vi "TranslateTyping.vi"(11 "Cluster":T2) -> (2 "key":string)   [LabVIEW 2020]
uses:
  <vilib>/event_ctls.llb/eventvkey.ctl
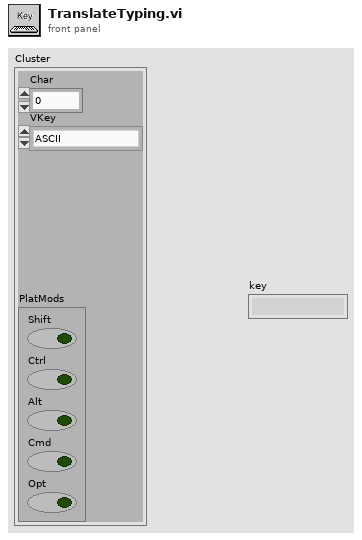
[diagram p1: front panel]
types:
  T1 = typedef "eventvkey.ctl" = enum16{"ASCII", "Enter", "Return", "Shift", "Ctrl", "Alt", "Cmd", "Opt", "Caps", "NumLock", "Clear", "Break", "Up", "Down", "Left", "Right", "Insert", "Delete", "Home", "End", "PageUp", "PageDown", "Escape", "Help", "Pause", "ScrollLock", "F1", "F2", "F3", "F4", "F5", "F6", "F7", "F8", "F9", "F10", "F11", "F12", "F13", "F14", "F15", "F16", "F17", "F18", "F19", "F20", "F21", "F22", "F23", "F24", "Play", "VolumeUp", "VolumeDown", "Mute", "Two Byte Char"}
  T2 = cluster{"Char":i16, "VKey":T1, "PlatMods":cluster{"Shift":bool, "Ctrl":bool, "Alt":bool, "Cmd":bool, "Opt":bool}}
  T3 = cluster{"Shift":bool, "Ctrl":bool, "Alt":bool, "Cmd":bool, "Opt":bool}
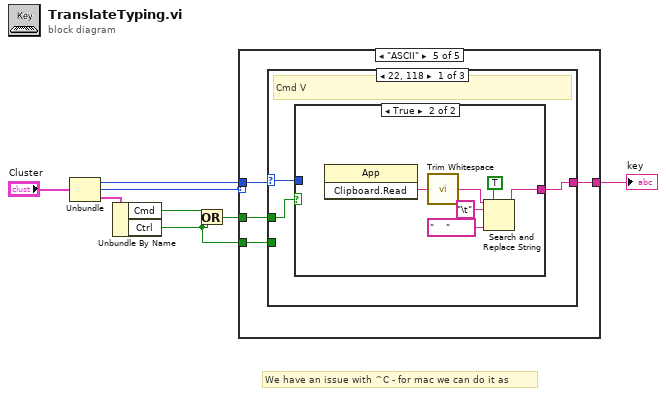
[diagram p0: block diagram]
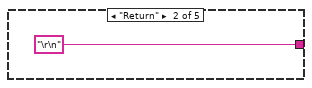
[diagram p3: hidden frame]
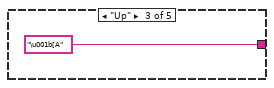
[diagram p4: hidden frame]
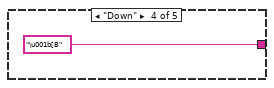
[diagram p5: hidden frame]
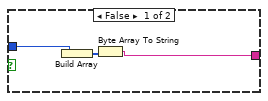
[diagram p6: hidden frame]
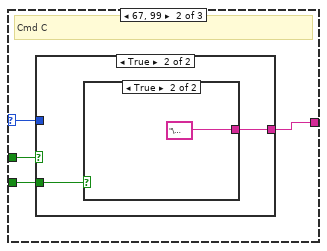
[diagram p7: hidden frame]
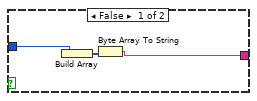
[diagram p8: hidden frame]
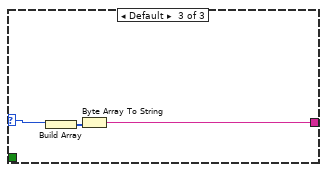
[diagram p10: hidden frame]
diagram:
  # "We have an issue with ^C - for mac we can do it as"
  n1 = Unbundle("Cluster") -> ("Char"=w7:i16, "VKey"=w6:T1, "PlatMods"=w1:T3)
  n2 = Unbundle By Name(w1) -> ("Cmd"=w3:bool, "Ctrl"=w5:bool)
  n3 = Or(x=w3, y=w5) -> (x .or. y?=w2:bool)
  n4 = case shown="\"ASCII\"" w6 {
    tunnel: [_ "\r\n" ("string") "\u001b[A" ("string") "\u001b[B" ("string") w15] -> w4
    tunnel: w7 -> [_ _ _ _ w14]
    tunnel: w2 -> [_ _ _ _ w13]
    tunnel: w5 -> [_ _ _ _ w12]
    frame Default {
    }
    frame "Return" {
    }
    frame "Up" {
    }
    frame "Down" {
    }
    frame "ASCII" {
      n5 = case shown="22, 118" w14 {
        selector: w14 -> [w16 w29 w38]
        tunnel: [w18 w31 w40] -> w15
        tunnel: w13 -> [w17 w30 _]
        tunnel: w12 -> [_ w28 _]
        frame 22, 118 {
          # "Cmd V"
          n6 = case shown="True" w17 {
            tunnel: [w19 w22] -> w18
            tunnel: w16 -> [w20 _]
            frame False {
              n7 = Build Array(w20) -> (w21:i16[])
              n8 = Byte Array To String(unsigned byte array=w21) -> (string=w19:string)
            }
            frame True {
              n9 = invoke class="App" method="Clipboard.Read"() -> ("Read Clipbrd"=w27:string)  [unwired: 3 in, 2 out]
              n10 = call <vilib>:"Trim Whitespace.vi"("string"=w27) -> ("trimmed string"=w26:string)  [unwired: 1 in]
              n11 = Search and Replace String(replace all?=TRUE ("replace all? (F)"), input string=w26, search string="\t", replace string="    " ("replace string (\"\")")) -> (result string=w22:string)  [unwired: 4 in, 3 out]
            }
          }
        }
        frame 67, 99 {
          # "Cmd C"
          n12 = case shown="True" w30 {
            tunnel: [w32 w35] -> w31
            tunnel: w29 -> [w33 _]
            tunnel: w28 -> [_ w36]
            frame False {
              n13 = Build Array(w33) -> (w34:i16[])
              n14 = Byte Array To String(unsigned byte array=w34) -> (string=w32:string)
            }
            frame True {
              n15 = case shown="True" w36 {
                tunnel: [_ "\u0003"] -> w35
                frame False {
                }
                frame True {
                }
              }
            }
          }
        }
        frame Default {
          n16 = Build Array(w38) -> (w39:i16[])
          n17 = Byte Array To String(unsigned byte array=w39) -> (string=w40:string)
        }
      }
    }
  }
  "key" <- w4
